vi "communication (SubVI).vi"(6 "Reset":bool, 7 "Data":bool, 9 "State":bool, 10 "file path (use dialog)":path=path "C:/tyrmt/data.csv.txt", 11 "VISA Refnum in":refnum<visa-resource-name>="COM4") -> (3 "State buffer":string)   [LabVIEW 2011]
uses:
  <vilib>/Instr/_visa.llb/VISA Configure Serial Port (Instr).vi
panel:
  out "stripped path":path
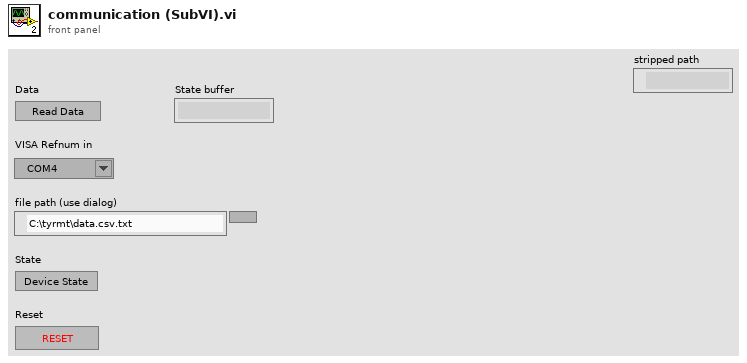
[diagram p1: front panel]
types:
  T1 = enum16{"open", "replace", "create", "open or create", "replace or create", "replace or create with confirmation"}
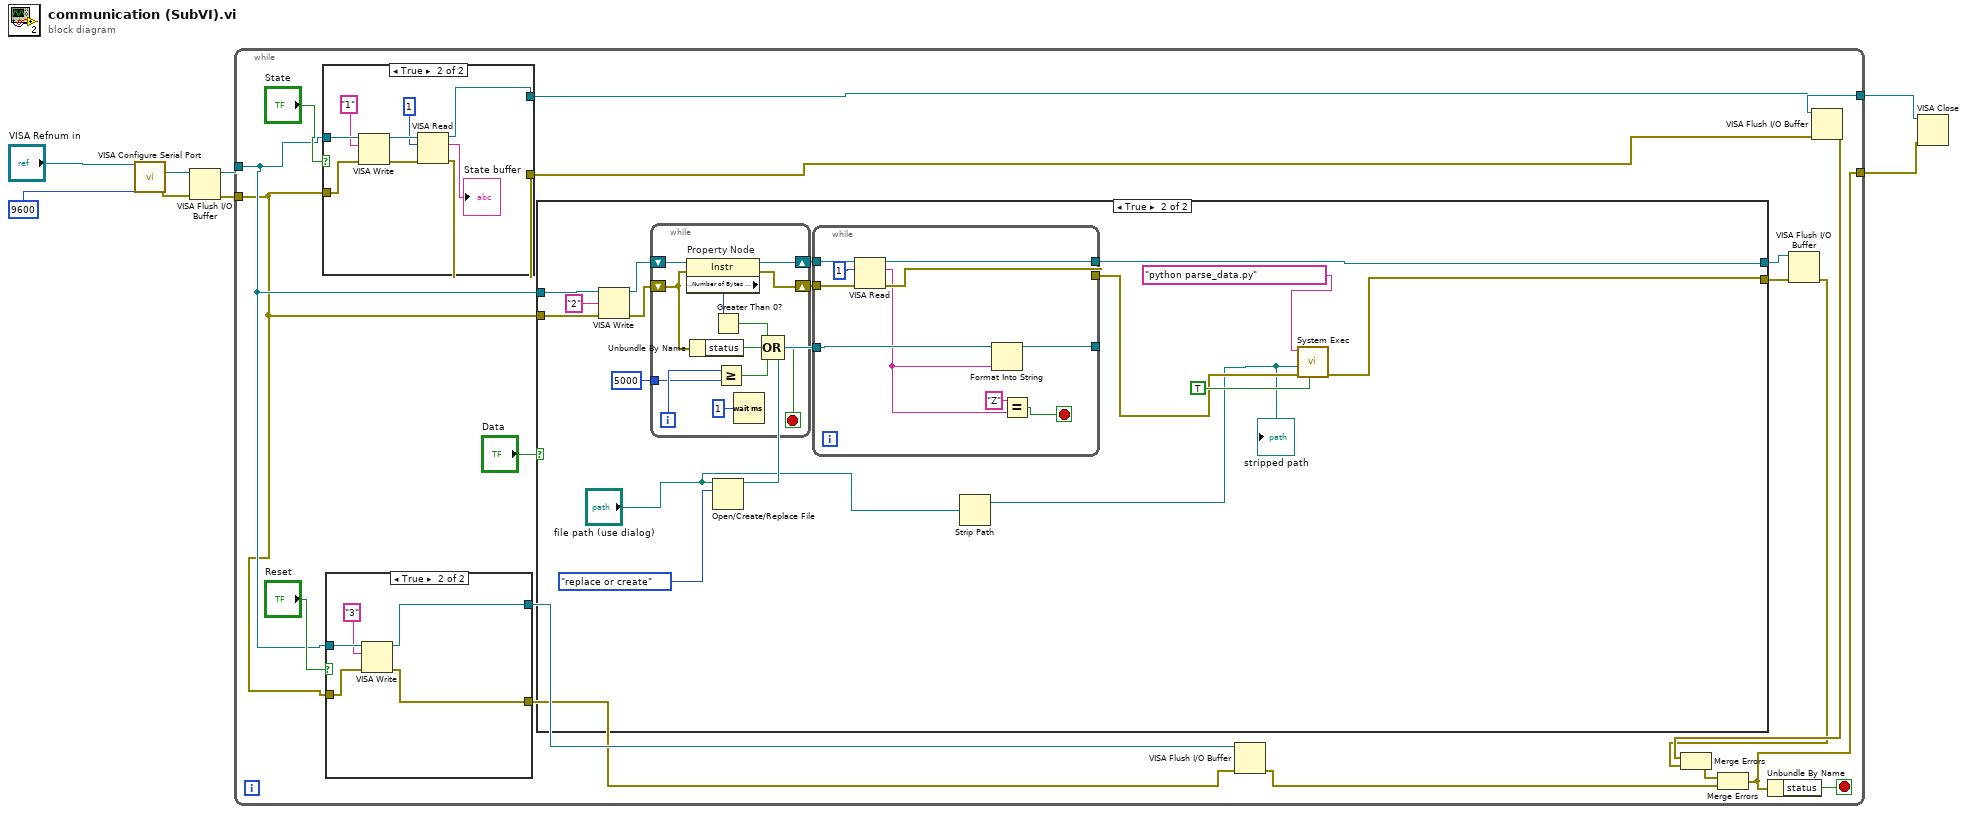
[diagram p0: block diagram]
diagram:
  n1 = call-poly "VISA Configure Serial Port"("VISA resource name"="VISA Refnum in", "baud rate (9600)"=9600) -> ("VISA resource name out"=w2:refnum<visa-resource-name>, "error out"=w3:errorcluster)  [unwired: 12 in]
  n2 = VISA Flush I/O Buffer(VISA resource name=w2, error in (no error)=w3) -> (VISA resource name out=w5:refnum<visa-resource-name>, error out=w6:errorcluster)  [unwired: 1 in]
  n3 = while {
    tunnel: w5 -> [w22]
    tunnel: w6 -> [w21]
    tunnel: [w11] -> w7
    tunnel: [w20] -> w8
    stop <- w24 stop-if-true
    n4 = case shown="True" "State" {
      tunnel: w22 -> [w76 w85]
      tunnel: w21 -> [w75 w84]
      tunnel: [w76 w79] -> w10
      tunnel: [w75 w78] -> w15
      frame False {
      }
      frame True {
        n5 = VISA Write(VISA resource name=w85, write buffer="1", error in (no error)=w84) -> (VISA resource name out=w81:refnum<visa-resource-name>, error out=w82:errorcluster)  [unwired: 1 out]
        n6 = VISA Read(VISA resource name=w81, byte count=1, error in (no error)=w82) -> (VISA resource name out=w79:refnum<visa-resource-name>, read buffer=→"State buffer":string, error out=w78:errorcluster)  [unwired: 1 out]
      }
    }
    n7 = case shown="True" "Reset" {
      tunnel: w22 -> [w69 w74]
      tunnel: w21 -> [w68 w73]
      tunnel: [w69 w71] -> w19
      tunnel: [w68 w70] -> w18
      frame False {
      }
      frame True {
        n8 = VISA Write(VISA resource name=w74, write buffer="3", error in (no error)=w73) -> (VISA resource name out=w71:refnum<visa-resource-name>, error out=w70:errorcluster)  [unwired: 1 out]
      }
    }
    n9 = case shown="True" "Data" {
      tunnel: w22 -> [w28 w45]
      tunnel: w21 -> [w27 w44]
      tunnel: [w28 w37] -> w16
      tunnel: [w27 w32] -> w14
      frame False {
      }
      frame True {
        n10 = VISA Write(VISA resource name=w45, write buffer="2", error in (no error)=w44) -> (VISA resource name out=w42:refnum<visa-resource-name>, error out=w41:errorcluster)  [unwired: 1 out]
        n11 = while {
          shift-right: [w66] -> w39
          shift-left: w42 -> [w67]
          shift-right: [w65] -> w38
          shift-left: w41 -> [w63]
          tunnel: 5000 ("Timeout (mS)") -> [w61]
          i -> [w62]
          stop <- w57 stop-if-true
          n12 = property on="Property Node" class="Instr"(reference=w67, error in=w63) -> (reference out=w66:refnum<visa-resource-name>, error out=w65:errorcluster, "Serial Settings:Number of Bytes at Serial Port"=w64:u32)
          n13 = Unbundle By Name(w63) -> ("status"=w59:bool)
          n14 = Greater Than 0?(x=w64) -> (x > 0?=w60:bool)
          n15 = Greater Or Equal?(x=w62, y=w61) -> (x >= y?=w58:bool)
          n16 = Wait (ms)(milliseconds to wait=u32 1) -> ()  [unwired: 1 out]
          n17 = Compound Arithmetic op=OR(w60, w59, w58) -> (w57:bool)
        }
        n18 = Open/Create/Replace File(file path (use dialog)="file path (use dialog)", operation (0:open)=T1."replace or create") -> (refnum out=w35:refnum<file>)  [unwired: 4 in, 2 out]
        n19 = while {
          tunnel: w39 -> [w54]
          tunnel: w38 -> [w55]
          tunnel: [w51] -> w37
          tunnel: [w50] -> w33
          tunnel: w35 -> [w48]
          tunnel: [w47] -> _
          stop <- w53 stop-if-true
          n20 = VISA Read(VISA resource name=w54, byte count=u32 1, error in (no error)=w55) -> (VISA resource name out=w51:refnum<visa-resource-name>, read buffer=w46:string, error out=w50:errorcluster)  [unwired: 1 out]
          n21 = Format Into String(initial string=w48, w46) -> (resulting string=w47:refnum<file>)  [unwired: 2 in, 1 out]
          n22 = Equal?(x="Z", y=w46) -> (x = y?=w53:bool)
        }
        n23 = Strip Path(path="file path (use dialog)") -> (stripped path=w29:path)  [unwired: 1 out]
        "stripped path" <- w29
        n24 = call <vilib>:"System Exec.vi"("run minimized? (F)"=TRUE, "error in (no error)"=w33, "working directory"=w29, "command line"="python parse_data.py") -> ("error out"=w32:errorcluster)  [unwired: 4 in, 3 out]
      }
    }
    n25 = VISA Flush I/O Buffer(VISA resource name=w19, error in (no error)=w18) -> (error out=w17:errorcluster)  [unwired: 1 in, 1 out]
    n26 = VISA Flush I/O Buffer(VISA resource name=w16, error in (no error)=w14) -> (error out=w9:errorcluster)  [unwired: 1 in, 1 out]
    n27 = VISA Flush I/O Buffer(VISA resource name=w10, error in (no error)=w15) -> (VISA resource name out=w11:refnum<visa-resource-name>, error out=w12:errorcluster)  [unwired: 1 in]
    n28 = Merge Errors(w12, w9) -> (w13:errorcluster)
    n29 = Merge Errors(w13, w17) -> (w20:errorcluster)
    n30 = Unbundle By Name(w20) -> ("status"=w24:bool)
  }
  n31 = VISA Close(VISA resource name=w7, error in (no error)=w8) -> ()  [unwired: 1 out]
